vi "Boot component.vi"(8 "error in (no error)":errorcluster, 10 "parameters":T1, 11 "ServiceManager in":refnum<class "ServiceManager.lvclass">) -> (0 "error out":errorcluster, 2 "component found?":bool, 3 "ServiceManager out":refnum<class "ServiceManager.lvclass">)   [LabVIEW 2012, in "ServiceManager.lvclass"]
uses:
  ServiceManager.lvclass
  boot_parameters_cluster.ctl
  Murmex/LabVIEW/Murmex/Murmex/component_specification_cluster.ctl
  <vilib>/Utility/file.llb/Read From Spreadsheet File (string).vi
  Murmex/LabVIEW/Murmex/Murmex/Murmex.lvclass
panel:
  out "All Files in Dir":path[](array[path])
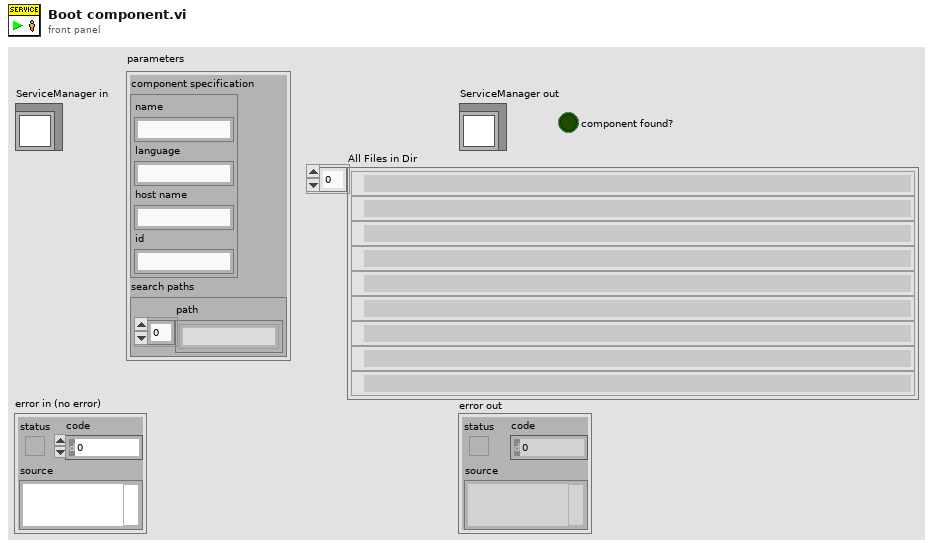
[diagram p1: front panel]
types:
  T1 = typedef "ServiceManager.lvclass/boot_parameters_cluster.ctl" = cluster{"component specification":T2, "search paths":cluster{"path":string[]}}
  T2 = typedef "Murmex.lvlib/Murmex.lvclass/component_specification_cluster.ctl" = cluster{"name":string, "language":string, "host name":string, "id":string}
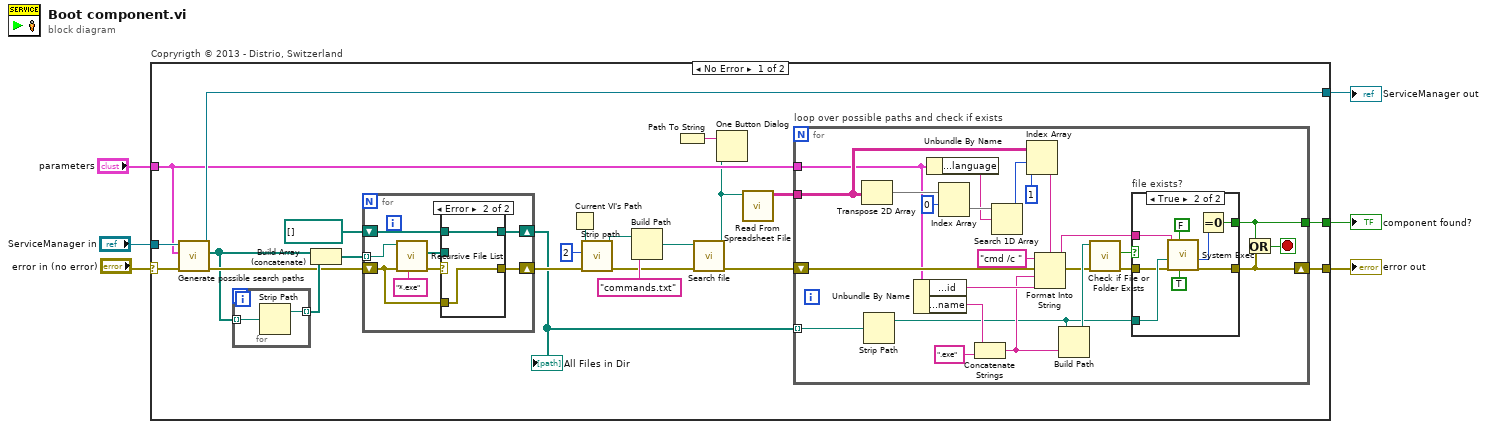
[diagram p0: block diagram]
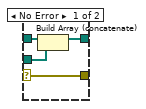
[diagram p2: hidden frame]
diagram:
  n1 = case "Copryrigth © 2013 - Distrio, Switzerland" shown="No Error" "error in (no error)" {
    selector: "error in (no error)" -> [w21 w81]
    tunnel: [w26 w81] -> w5
    tunnel: [w19 w80] -> w4
    tunnel: "ServiceManager in" -> [w20 w80]
    tunnel: "parameters" -> [w18 _]
    tunnel: [w27 _] -> w1
    frame No Error {
      n2 = call-dynamic "Generate possible search paths.vi"("error in (no error)"=w21, "parameters"=w18, "ServiceManager in"=w20) -> ("error out"=w15:errorcluster, "path array out"=w11:path[], "ServiceManager out"=w19:refnum<class "ServiceManager.lvclass">)  [unwired: 6 in]
      n3 = for {
        tunnel: w11 -> [w45] mode=indexing
        tunnel: [w44] -> w17 mode=indexing
        n4 = Strip Path(path=w45) -> (stripped path=w44:path)  [unwired: 1 out]
      }
      n5 = Build Array (concatenate)(w11, w17) -> (w10:path[])
      n6 = for {
        tunnel: w10 -> [w37] mode=indexing
        shift-right: [w34] -> w13
        shift-left: path[] [] ("All Files in Dir") -> [w36]
        shift-right: [w31] -> w14
        shift-left: w15 -> [w30]
        n7 = call <vilib>:"Recursive File List.vi"("pattern"="*.exe" ("string"), "error in (no error)"=w30, "Folder Path"=w37) -> ("error out"=w32:errorcluster, "All Files in Dir"=w35:path[])  [unwired: 4 in, 3 out]
        n8 = case shown="Error" w32 {
          selector: w32 -> [w38 _]
          tunnel: w36 -> [w41 w43]
          tunnel: w35 -> [w40 _]
          tunnel: [w39 w43] -> w34
          tunnel: [w38 w42] -> w31
          tunnel: w30 -> [_ w42]
          frame No Error {
            n9 = Build Array (concatenate)(w41, w40) -> (w39:path[])
          }
          frame Error {
          }
        }
      }
      "All Files in Dir" <- w13
      n10 = Current VI's Path() -> (path=w24:path)
      n11 = call "Strip path.vi"("error in (no error)"=w14, "number of strips"=2, "path in"=w24) -> ("error out"=w25:errorcluster, "path out"=w22:path)  [unwired: 7 in]
      n12 = Build Path(base path=w22, name or relative path="commands.txt") -> (appended path=w9:path)
      n13 = call "Search file.vi"("error in (no error)"=w25, "path in"=w9) -> ("error out"=w12:errorcluster, "path out"=w7:path)  [unwired: 7 in, 1 out]
      n14 = Path To String(path=w7) -> (string=w8:string)
      n15 = One Button Dialog(message=w8) -> ()  [unwired: 1 in, 1 out]
      n16 = call-poly <vilib>:"Read From Spreadsheet File.vi"("file path (dialog if empty)"=w7) -> ("all rows"=w29:string[][])  [unwired: 6 in, 4 out]
      n17 = for "loop over possible paths and check if exists" {
        tunnel: w29 -> [w66]
        tunnel: w18 -> [w60]
        tunnel: w13 -> [w47] mode=indexing
        tunnel: [w55] -> w27
        shift-right: [w57] -> w26
        shift-left: w12 -> [w61]
        stop <- w56 stop-if-true
        n18 = Transpose 2D Array(2D array=w66) -> (transposed array=w70:string[][])
        n19 = Strip Path(path=w47) -> (stripped path=w46:path)  [unwired: 1 out]
        n20 = Unbundle By Name(w60) -> ("component specification.id"=w62:string, "component specification.name"=w49:string)
        n21 = Unbundle By Name(w60) -> ("component specification.language"=w67:string)
        n22 = Index Array(array=w70, index (row)=0) -> (element=w68:string[])  [unwired: 1 in]
        n23 = Concatenate Strings(w49, ".exe" ("string")) -> (w50:string)
        n24 = Search 1D Array(1D array=w68, element=w67) -> (index of element=w65:i32)  [unwired: 1 in]
        n25 = Index Array(array=w66, index (row)=w65, index (col)=1 ("disabled index (col)")) -> (element=w59:string)
        n26 = Format Into String(format string=w59, initial string="cmd /c ", error in=w61, w50, w62) -> (resulting string=w58:string, error out=w52:errorcluster)
        n27 = Build Path(base path=w46, name or relative path=w50) -> (appended path=w53:path)
        n28 = call <vilib>:"Check if File or Folder Exists.vi"("error in (no error)"=w52, "path"=w53) -> ("error out"=w51:errorcluster, "file or folder exists?"=w48:bool)  [unwired: 7 in, 1 out]
        n29 = case "file exists?" shown="True" w48 {
          tunnel: w58 -> [_ w77]
          tunnel: [w71 w75] -> w57
          tunnel: [_ w74] -> w55
          tunnel: w46 -> [_ w73]
          tunnel: w51 -> [w71 w72]
          frame False {
          }
          frame True {
            n30 = call <vilib>:"System Exec.vi"("run minimized? (F)"=TRUE, "wait until completion? (T)"=FALSE, "error in (no error)"=w72, "working directory"=w73, "command line"=w77) -> ("error out"=w75:errorcluster, "return code"=w76:i32)  [unwired: 3 in, 2 out]
            n31 = Equal To 0?(x=w76) -> (x = 0?=w74:bool)
          }
        }
        n32 = Or(x=w55, y=w57) -> (x .or. y?=w56:bool)
      }
    }
    frame Error {
    }
  }
  "error out" <- w5
  "ServiceManager out" <- w4
  "component found?" <- w1
